vi "Scope_D2.vi"   [LabVIEW 2019]
uses:
  <userlib>/_TI-LA/Instr Drivers/Oscilloscope/MSO5X/Driver/Base/Tektronix MSO5X Series.lvlib
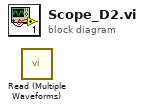
[diagram p0: block diagram]
diagram:
  n1 = call <userlib>:"Read (Multiple Waveforms).vi"() -> ()  [unwired: 9 in, 3 out]
